vi "ListMFCchannels.vi"(7 "Channel names set":T1, 11 "Gas Release System":string) -> (0 "C2H6descriptions":T2[](array[typedef]) {"mDot" format="%_4g"; "Setpoint" format="%.2g"; "MFCcapability"."MaxMdot" format="%_4g"; "MFCcapability"."MinMdot" format="%_4g"}, 1 "N2descriptions":T2[](array[typedef]) {"mDot" format="%_4g"; "Setpoint" format="%.2g"; "MFCcapability"."MaxMdot" format="%_4g"; "MFCcapability"."MinMdot" format="%_4g"})   [LabVIEW 2021]
uses:
  MFCdescription.ctl
  MFCcapability.ctl
  ADAM Client/Sub VIs/ADAM Controls/Channel_names.ctl
panel:
  out "message":string
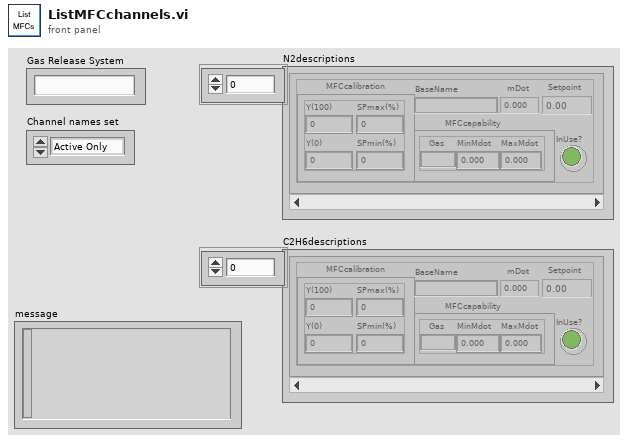
[diagram p1: front panel]
types:
  T1 = typedef "Channel_names.ctl" = enum16{"Active Only", "Active + Off", "All Channels"}
  T2 = typedef "MFCdescription.ctl" = cluster{"BaseName":string, "MFCcalibration":cluster{"Y(100)":dbl, "Y(0)":dbl, "SPmin(%)":dbl, "SPmax(%)":dbl}, "MFCcapability":T3, "InUse?":bool, "Setpoint":dbl, "mDot":dbl}
  T3 = typedef "MFCcapability.ctl" = cluster{"Gas":string, "MinMdot":dbl, "MaxMdot":dbl}
  T4 = typedef "Ch_description_ADAM.ctl" = cluster{"Ch Name":string, "Type":T5, "Function":T6, "Ch State":T7, "Calibration type":T8, "A":dbl, "B":dbl, "C":dbl, "D":dbl, "Comments":string, "Address":T9, "String":string, "Duty":u16}
  T5 = typedef "Module_type_ADAM.ctl" = string
  T6 = typedef "Function_ADAM.ctl" = enum16{"Analogue Input", "Digital Input", "Event counter", "Event rate", "Analogue Output", "Digital Output", "Relay Output"}
  T7 = typedef "Channel_State.ctl" = enum16{"On", "Off", "Always On", "Always Off"}
  T8 = typedef "Calib_type_ADAM.ctl" = string
  T9 = typedef "Address.ctl" = cluster{"Main":i32, "Ch.":i32, "Sub":i32, "Port Name":string}
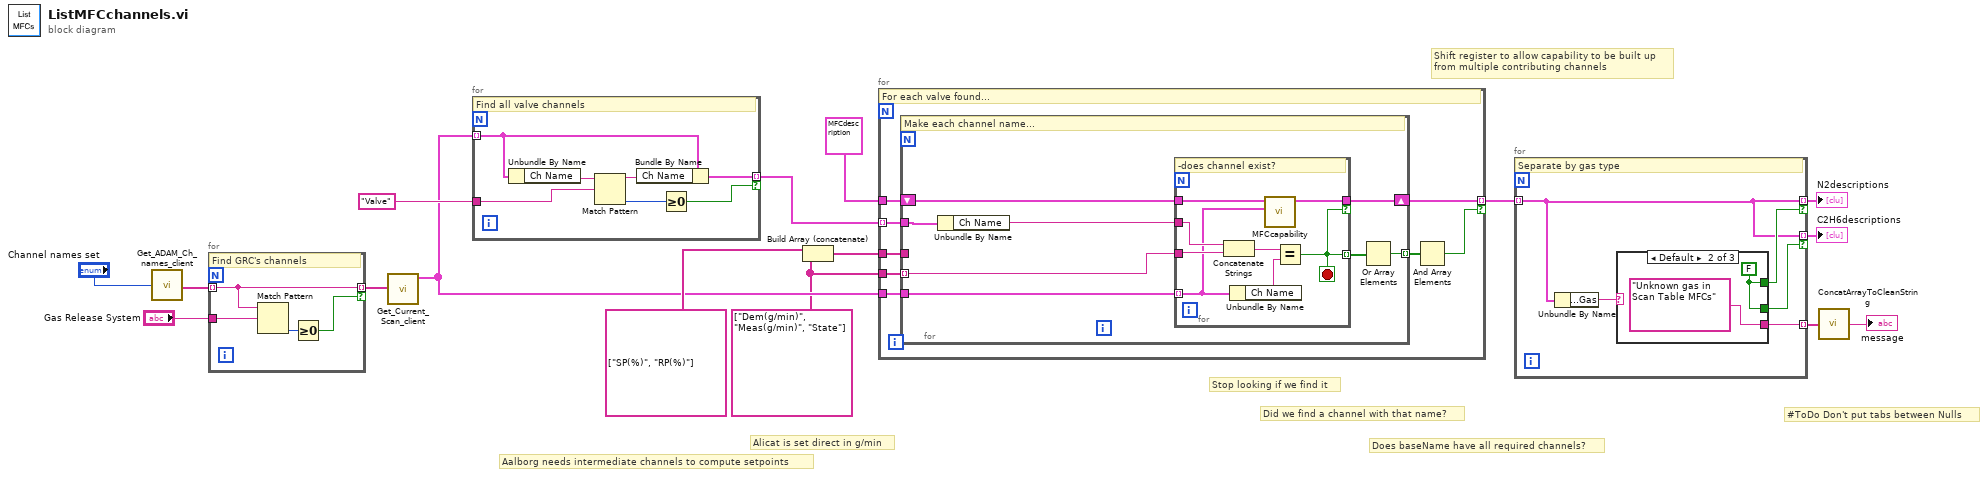
[diagram p0: block diagram]
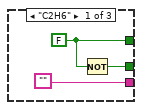
[diagram p2: hidden frame]
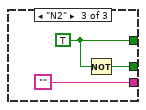
[diagram p3: hidden frame]
diagram:
  w1 = string[] ["Dem(g/min)", "Meas(g/min)", "State"]
  # "Alicat is set direct in g/min"
  # "Shift register to allow capability to be built up from multiple contributing channels"
  # "Stop looking if we find it"
  # "Did we find a channel with that name?"
  # "Does baseName have all required channels?"
  # "#ToDo Don't put tabs between Nulls"
  # "Aalborg needs intermediate channels to compute setpoints"
  n1 = call "Get_ADAM_Ch_names_client.vi"("Channel names set"="Channel names set") -> ("Ch names"=w3:string[])
  n2 = for {
    tunnel: w3 -> [w18] mode=indexing
    tunnel: "Gas Release System" -> [w20]
    tunnel: [w18] -> w6 mode=indexing if=w17
    # "Find GRC's channels"
    n3 = Match Pattern(string=w18, regular expression=w20) -> (offset past match=w19:i32)  [unwired: 1 in, 3 out]
    n4 = Greater Or Equal To 0?(x=w19) -> (x >= 0?=w17:bool)
  }
  n5 = call "Get_Current_Scan_client.vi"("multipleChannels"=w6) -> ("Ch Description Array"=w5:T4[])  [unwired: 1 in, 3 out]
  n6 = for {
    tunnel: w5 -> [w24] mode=indexing
    tunnel: [w22] -> w12 mode=indexing if=w25
    tunnel: "Valve" -> [w21]
    # "Find all valve channels"
    n7 = Unbundle By Name(w24) -> ("Ch Name"=w26:string)
    n8 = Match Pattern(string=w26, regular expression=w21) -> (before substring=w23:string, offset past match=w27:i32)  [unwired: 1 in, 2 out]
    n9 = Bundle By Name(cluster=w24, "Ch Name"=w23) -> (w22:T4)
    n10 = Greater Or Equal To 0?(x=w27) -> (x >= 0?=w25:bool)
  }
  n11 = Build Array (concatenate)(string[] ["SP(%)", "RP(%)"], w1) -> (w2:string[])
  n12 = for {
    tunnel: w12 -> [w35] mode=indexing
    tunnel: w2 -> [w34]
    tunnel: w5 -> [w33]
    tunnel: [w31] -> w9 mode=indexing if=w30
    tunnel: T2 {"BaseName"="Error", "MFCcalibration"={"Y(100)"=0.0, "Y(0)"=0.0, "SPmin(%)"=0.0, "SPmax(%)"=0.0}, "MFCcapability"={"Gas"="", "MinMdot"=0.0, "MaxMdot"=0.0}, "InUse?"=FALSE, "Setpoint"=0.0, "mDot"=0.0} ("MFCdescriptionOut") -> [w29]
    tunnel: w1 -> [w28]
    # "For each valve found..."
    n13 = for {
      tunnel: w35 -> [w43]
      tunnel: w34 -> [_]
      tunnel: w33 -> [w42]
      tunnel: [w40] -> w32 mode=indexing
      shift-right: [w39] -> w31
      shift-left: w29 -> [w38]
      tunnel: w28 -> [w36] mode=indexing
      # "Make each channel name..."
      n14 = Unbundle By Name(w43) -> ("Ch Name"=w37:string)
      n15 = for {
        tunnel: w42 -> [w47] mode=indexing
        tunnel: w36 -> [w48]
        tunnel: [w46] -> w41 mode=indexing
        tunnel: w37 -> [w49]
        tunnel: [w44] -> w39 if=w46
        tunnel: w38 -> [w45]
        stop <- w46 stop-if-true
        # "-does channel exist?"
        n16 = Concatenate Strings(w49, w48) -> (w50:string)
        n17 = Unbundle By Name(w47) -> ("Ch Name"=w51:string)
        n18 = call "MFCcapability.vi"("Ch Description"=w47, "MFCdescriptionIn"=w45) -> ("MFCdescriptionOut"=w44:T2)  [unwired: 9 in]
        n19 = Equal?(x=w50, y=w51) -> (x = y?=w46:bool)
      }
      n20 = Or Array Elements(Boolean array=w41) -> (logical OR=w40:bool)
    }
    n21 = And Array Elements(Boolean array=w32) -> (logical AND=w30:bool)
  }
  n22 = for {
    tunnel: [w53] -> w15 mode=indexing if=w55
    tunnel: [w53] -> w14 mode=indexing if=w54
    tunnel: w9 -> [w53] mode=indexing
    tunnel: [w52] -> w8 mode=indexing
    # "Separate by gas type"
    n23 = Unbundle By Name(w53) -> ("MFCcapability.Gas"=w56:string)
    n24 = case shown="Default" w56 {
      tunnel: [w59 w61 w64] -> w55
      tunnel: [w58 w61 w63] -> w54
      tunnel: ["" "Unknown gas in Scan Table MFCs" ("message") ""] -> w52
      frame "C2H6" {
        w59 = FALSE
        n25 = Not(x=w59) -> (.not. x?=w58:bool)
      }
      frame Default {
        w61 = FALSE
      }
      frame "N2" {
        w64 = TRUE
        n26 = Not(x=w64) -> (.not. x?=w63:bool)
      }
    }
  }
  "N2descriptions" <- w15
  "C2H6descriptions" <- w14
  n27 = call "ConcatArrayToCleanString.vi"("stringArray"=w8) -> ("cleanDelimitedString"=→"message":string)  [unwired: 1 in]
